vi "Varient_number_check.vi"(0 "Varient No.":u16, 5 "Varient path":path, 11 "error in":errorcluster) -> (1 "HARNESS_CODE":string, 2 "TORISHI_CODE":string, 4 "Part Name":string, 6 "Varient Number":i32, 8 "STATION 1 BYPASS":bool, 10 "Batch Size":i32, 12 "MODEL LIST":string[](array[string]), 14 "PART_NO":string, 15 "error out":errorcluster)   [LabVIEW 2017]
uses:
  <vilib>/Utility/config.llb/Read Key (I32).vi
  <vilib>/Utility/config.llb/Read Key (String).vi
  <vilib>/Utility/config.llb/Read Key (Boolean).vi
  <vilib>/Utility/config.llb/NI_LVConfig.lvlib
panel:
  # "Varient no. check"
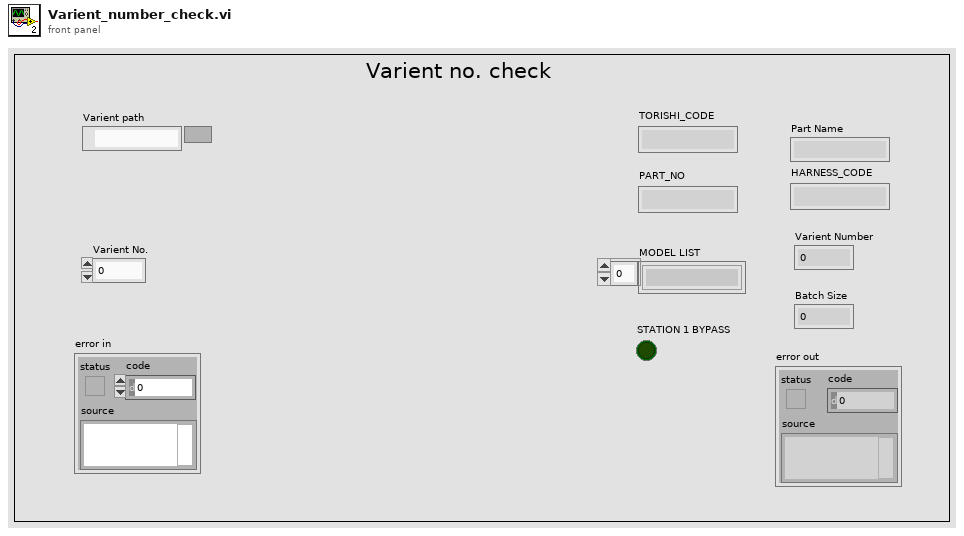
[diagram p1: front panel]
types:
  T1 = typedef "NI_LVConfig.lvlib/Config Data RefNum.ctl" = refnum<k1>
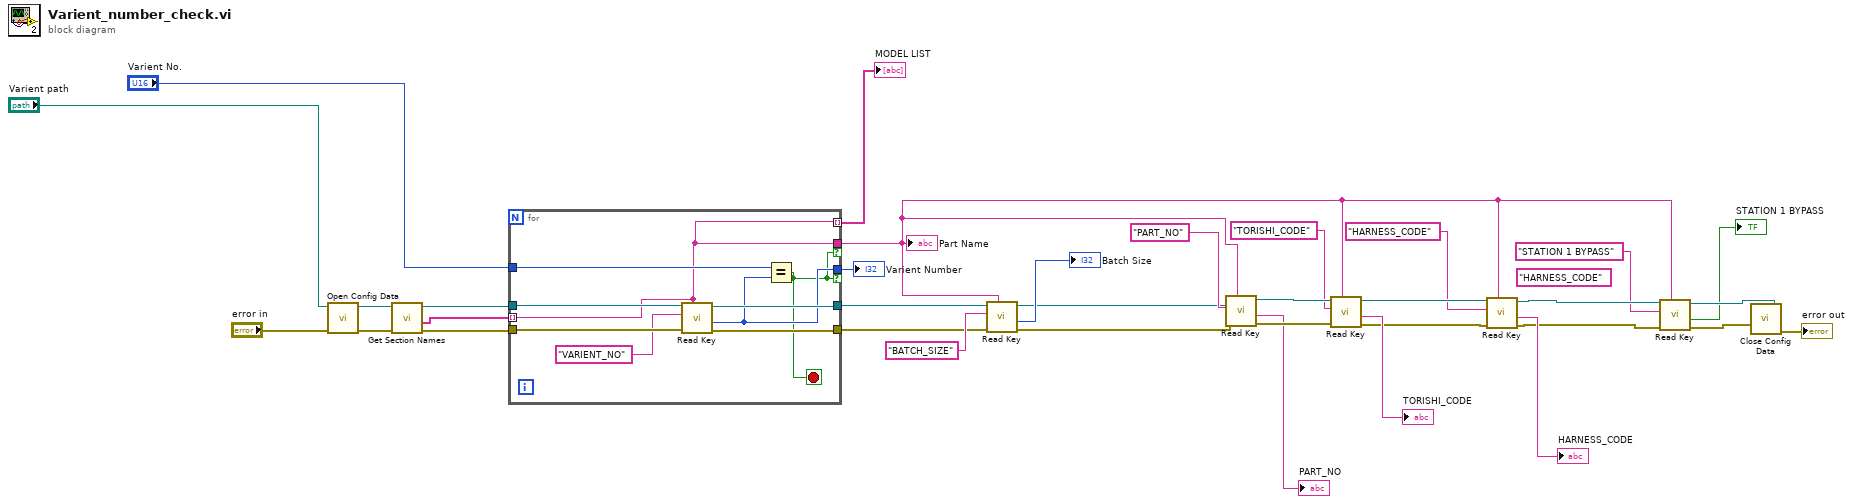
[diagram p0: block diagram]
diagram:
  (unwired) "HARNESS_CODE" ("key")
  n1 = call <vilib>:"Open Config Data.vi"("error in (no error)"="error in", "configuration file path"="Varient path") -> ("error out"=w33:errorcluster, "refnum"=w34:T1)  [unwired: 7 in, 1 out]
  n2 = call <vilib>:"Get Section Names.vi"("error in (no error)"=w33, "refnum"=w34) -> ("error out"=w30:errorcluster, "section names"=w28:string[], "refnum out"=w29:T1)  [unwired: 7 in]
  n3 = for {
    tunnel: w28 -> [w35] mode=indexing
    tunnel: w29 -> [w41]
    tunnel: [w40] -> w23
    tunnel: w30 -> [w43]
    tunnel: [w42] -> w24
    tunnel: [w37] -> w26 if=w36
    tunnel: "Varient No." -> [w38]
    tunnel: [w35] -> w3 if=w36
    tunnel: [w35] -> w12 mode=indexing
    stop <- w36 stop-if-true
    n4 = call-poly <vilib>:"Read Key.vi"("section"=w35, "error in (no error)"=w43, "key"="VARIENT_NO" ("name or relative path"), "refnum"=w41) -> ("error out"=w42:errorcluster, "value"=w37:i32, "refnum out"=w40:T1)  [unwired: 4 in, 1 out]
    n5 = Equal?(x=w38, y=w37) -> (x = y?=w36:bool)
  }
  "Varient Number" <- w26
  "Part Name" <- w3
  "MODEL LIST" <- w12
  n6 = call-poly <vilib>:"Read Key.vi"("section"=w3, "error in (no error)"=w24, "key"="BATCH_SIZE" ("name or relative path"), "refnum"=w23) -> ("error out"=w16:errorcluster, "value"=→"Batch Size":i32, "refnum out"=w17:T1)  [unwired: 4 in, 1 out]
  n7 = call-poly <vilib>:"Read Key.vi"("section"=w3, "error in (no error)"=w16, "key"="PART_NO", "refnum"=w17) -> ("error out"=w20:errorcluster, "value"=→"PART_NO":string, "refnum out"=w21:T1)  [unwired: 4 in, 1 out]
  n8 = call-poly <vilib>:"Read Key.vi"("section"=w3, "error in (no error)"=w20, "key"="TORISHI_CODE", "refnum"=w21) -> ("error out"=w10:errorcluster, "value"=→"TORISHI_CODE":string, "refnum out"=w9:T1)  [unwired: 4 in, 1 out]
  n9 = call-poly <vilib>:"Read Key.vi"("section"=w3, "error in (no error)"=w10, "key"="HARNESS_CODE", "refnum"=w9) -> ("error out"=w7:errorcluster, "value"=→"HARNESS_CODE":string, "refnum out"=w5:T1)  [unwired: 4 in, 1 out]
  n10 = call-poly <vilib>:"Read Key.vi"("section"=w3, "error in (no error)"=w7, "key"="STATION 1 BYPASS", "refnum"=w5) -> ("error out"=w6:errorcluster, "value"=→"STATION 1 BYPASS":bool, "refnum out"=w4:T1)  [unwired: 4 in, 1 out]
  n11 = call <vilib>:"Close Config Data.vi"("error in (no error)"=w6, "refnum"=w4) -> ("error out"=→"error out":errorcluster)  [unwired: 8 in, 1 out]
